vi "CreateListener.vi"(8 "error in (no error)":errorcluster, 11 "qbus in":refnum<class "Qbus.lvclass">) -> (0 "error out":errorcluster, 3 "qbus out":refnum<class "Qbus.lvclass">)   [LabVIEW 2015, in "DeleteProcess.lvlib"]
doc: "Integrates the Timer process with the Qbus message bus."
uses:
  DeleteProcess.lvlib
  <vilib>/addons/Qbus/Qbus.lvclass
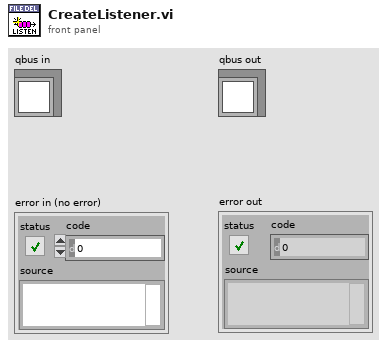
[diagram p1: front panel]
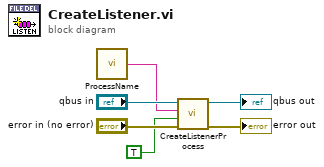
[diagram p0: block diagram]
diagram:
  n1 = call "ProcessName.vi"() -> ("process name"=w2:string)  [unwired: 5 in]
  n2 = call <vilib>:"CreateListenerProcess.vi"("error in (no error)"="error in (no error)", "master"=TRUE, "process name"=w2, "Qbus in"="qbus in") -> ("error in (no error)"=→"error out":errorcluster, "Qbus out"=→"qbus out":refnum<class "Qbus.lvclass">)  [unwired: 6 in]
